vi "Display FI locations on tiled image.vi"(5 "[user-specified font]":T1={"Font Name:"="", "Size"=8, "Strikeout?"=FALSE, "Italic?"=FALSE, "Underline?"=FALSE, "Outline?"=FALSE, "Shadow?"=FALSE, "Bold?"=FALSE}, 6 "Symbol":string="+", 7 "Primary grid @ green":bool=TRUE, 8 "Tiled Image fit to":u8(ring) items=["Width", "Height"], 9 "Focus Index Options":T2={"Keep aspect ratio"=FALSE, "Show Focus Index"=TRUE, "Focus Index primary grid center"=TRUE, "X Grids"=[[1]], "Y Grids"=[[1]], "Primary X index"=[[1]], "Primary Y index"=[[1]]} {"Y Grids" step=2; "X Grids" step=2}, 10 "SEM Scan Parameters":T3={"X size (um)"=80.0, "Y size (um)"=80.0, "X center (um)"=0.0, "Y center (um)"=0.0, "X size (V)"=3.7333333333333334, "X size auto"=TRUE, "X stig"=[[0.0]], "Y stig"=[[0.0]], "X aln"=[[0.0]], "Y aln"=[[0.0]], "Scan rate (Hz)"=10000000, "Oversampling"=5, "Oversampling auto"=TRUE, "Frame line rampdown ratio"=0.1, "Pixel size (nm)"=8.0, "WD (mm)"=[[3.0]], "X tiles"=1, "Y tiles"=1, "Overlap (um)"=2.0, "Interlaced"=TRUE, "dX (um)"=[0.0], "dY (um)"=[0.0], "Frames"=1} {"dY (um)" format="%.1f"; "dX (um)" format="%.1f"; "Frames" min=1 step=1; "WD (mm)" step=0.001 format="%.4f"; "Y aln" format="%.1f"; "X aln" format="%.1f"; "Y stig" format="%.1f"; "X stig" format="%.1f"; "Overlap (um)" min=0; "Y tiles" min=1; "X tiles" min=1; "X size (um)" format="%.2f"; "Y size (um)" format="%.2f"; "Frame line rampdown ratio" min=0 max=1 step=0.05 format="%.2g"; "X center (um)" step=1 format="%.3f"; "Y center (um)" step=1 format="%.3f"; "X size (V)" format="%_4g"; "Scan rate (Hz)" max=4000000 step=100000 format="%.2e"}, 11 "Image reference":refnum<vi>) -> ()   [LabVIEW 2018]
panel:
  # "Grids"
  # "Primary"
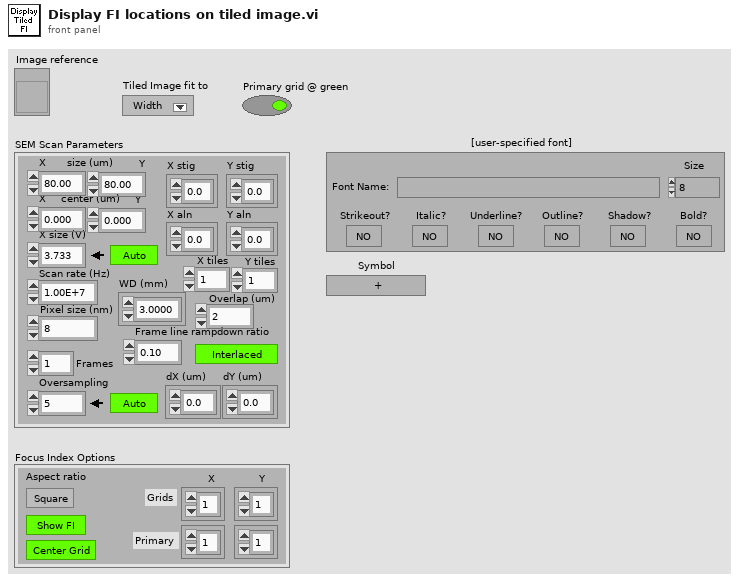
[diagram p1: front panel]
types:
  T1 = cluster{"Font Name:":string, "Size":i16, "Strikeout?":bool, "Italic?":bool, "Underline?":bool, "Outline?":bool, "Shadow?":bool, "Bold?":bool}
  T2 = cluster{"Keep aspect ratio":bool, "Show Focus Index":bool, "Focus Index primary grid center":bool, "X Grids":u8[][], "Y Grids":u8[][], "Primary X index":u8[][], "Primary Y index":u8[][]}
  T3 = cluster{"X size (um)":sgl, "Y size (um)":sgl, "X center (um)":sgl, "Y center (um)":sgl, "X size (V)":dbl, "X size auto":bool, "X stig":sgl[][], "Y stig":sgl[][], "X aln":sgl[][], "Y aln":sgl[][], "Scan rate (Hz)":u32, "Oversampling":u32, "Oversampling auto":bool, "Frame line rampdown ratio":sgl, "Pixel size (nm)":sgl, "WD (mm)":sgl[][], "X tiles":u8, "Y tiles":u8, "Overlap (um)":sgl, "Interlaced":bool, "dX (um)":sgl[], "dY (um)":sgl[], "Frames":u8}
  T4 = cluster{"horizontal":enum16{"left", "center", "right"}, "vertical":enum16{"top", "center", "bottom"}}
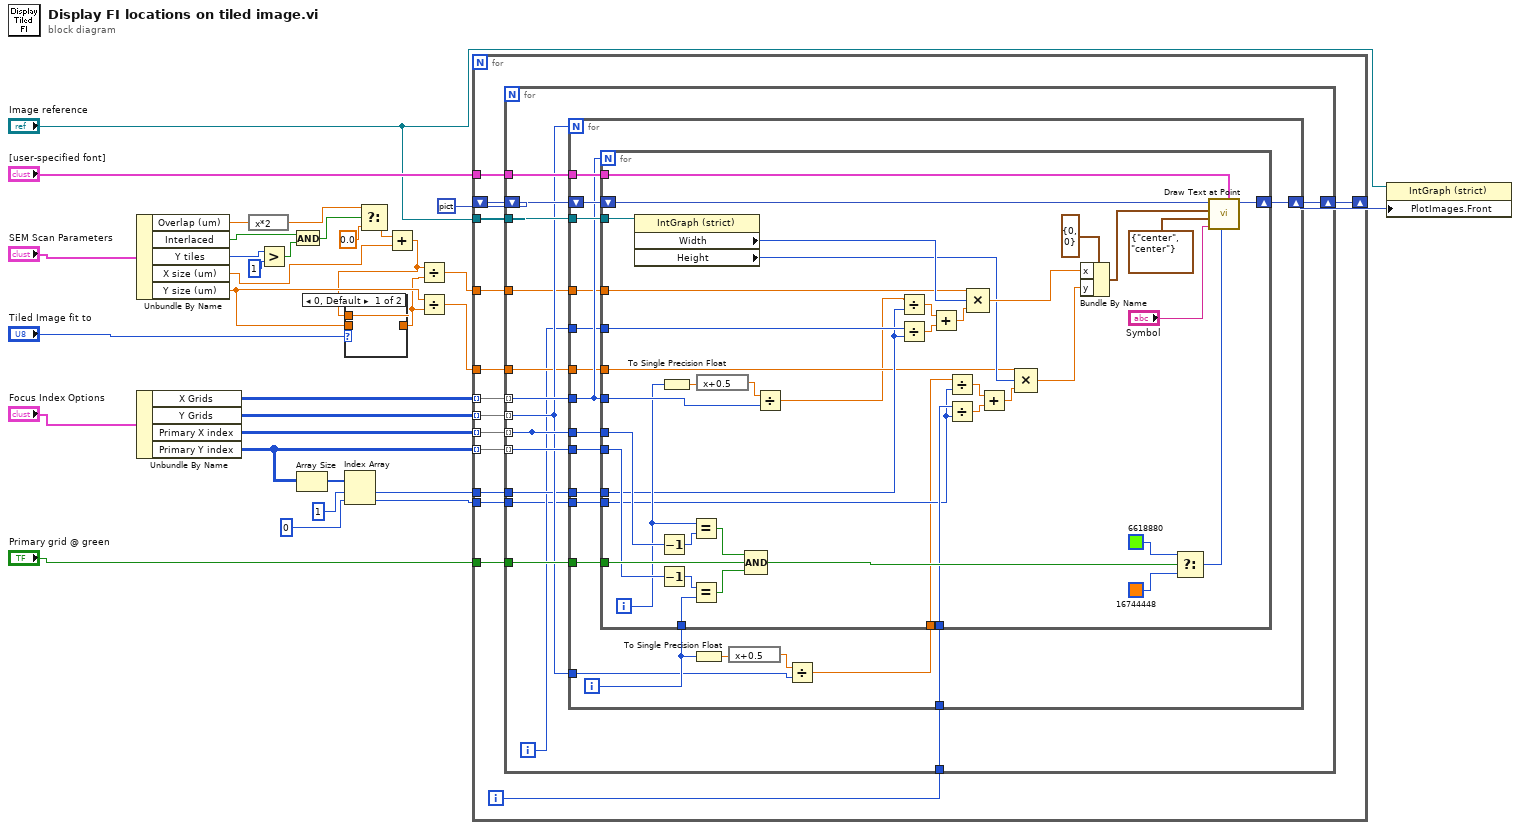
[diagram p0: block diagram]
diagram:
  n1 = Unbundle By Name("SEM Scan Parameters") -> ("Overlap (um)"=w7:sgl, "Interlaced"=w2:bool, "Y tiles"=w5:u8, "X size (um)"=w11:sgl, "Y size (um)"=w23:sgl)
  n2 = Unbundle By Name("Focus Index Options") -> ("X Grids"=w30:u8[][], "Y Grids"=w29:u8[][], "Primary X index"=w27:u8[][], "Primary Y index"=w16:u8[][])
  n3 = expression code="x*2"(w7) -> (w8:sgl)
  n4 = Greater?(x=w5, y=u8 1) -> (0:w3:bool)
  n5 = And(x=w2, y=w3) -> (x .and. y?=w1:bool)
  n6 = Array Size(array=w16) -> (size(s)=w17:i32[])
  n7 = Index Array(array=w17, index #1=1 ("index"), index #2=0 ("index")) -> (element #1=w15:i32, element #2=w14:i32)
  n8 = Select(t=w8, s=w1, f=0.0) -> (s? t:f=w10:dbl)
  n9 = Add(x=w10, y=w11) -> (x+y=w6:dbl)
  n10 = case shown="0, Default" "Tiled Image fit to" {
    tunnel: w6 -> [w33 _]
    tunnel: w23 -> [_ w34]
    tunnel: [w33 w34] -> w22
    frame 0, Default {
    }
    frame 1 {
    }
  }
  n11 = Divide(x=w6, y=w22) -> (x/y=w21:dbl)
  n12 = Divide(x=w23, y=w22) -> (x/y=w20:dbl)
  n13 = for {
    tunnel: w30 -> [w48] mode=indexing
    tunnel: w29 -> [w47] mode=indexing
    tunnel: "Image reference" -> [w46]
    shift-right: [w45] -> w13
    shift-left: picture data[5B] ("picture") -> [w44]
    tunnel: w27 -> [w43] mode=indexing
    tunnel: w16 -> [w42] mode=indexing
    tunnel: "[user-specified font]" -> [w41]
    tunnel: "Primary grid @ green" -> [w40]
    tunnel: w21 -> [w39]
    tunnel: w20 -> [w38]
    tunnel: w15 -> [w37]
    tunnel: w14 -> [w36]
    i -> [w35]
    n14 = for {
      tunnel: w48 -> [w63] mode=indexing
      tunnel: w47 -> [w55] mode=indexing
      tunnel: w46 -> [w62]
      shift-right: [w61] -> w45
      shift-left: w44 -> [w60]
      tunnel: [w57] -> _ mode=indexing
      tunnel: w43 -> [w57] mode=indexing
      tunnel: w42 -> [w56] mode=indexing
      tunnel: w41 -> [w59]
      tunnel: w40 -> [w58]
      tunnel: w39 -> [w54]
      tunnel: w38 -> [w53]
      tunnel: w37 -> [w52]
      tunnel: w36 -> [w50]
      tunnel: w35 -> [w49]
      i -> [w51]
      n15 = for {
        N: w55 -> [_]
        tunnel: w63 -> [w71]
        tunnel: w62 -> [w82]
        shift-right: [w81] -> w61
        shift-left: w60 -> [w80]
        tunnel: w59 -> [w79]
        tunnel: w58 -> [w78]
        tunnel: w57 -> [w77]
        tunnel: w56 -> [w76]
        tunnel: w55 -> [w72]
        tunnel: w54 -> [w70]
        tunnel: w53 -> [w68]
        tunnel: w52 -> [w67]
        tunnel: w51 -> [w66]
        tunnel: w50 -> [w65]
        tunnel: w49 -> [w64]
        i -> [w73]
        n16 = To Single Precision Float(number=w73) -> (single precision float=w74:sgl)
        n17 = expression code="x+0.5"(w74) -> (w75:sgl)
        n18 = Divide(x=w75, y=w72) -> (x/y=w69:sgl)
        n19 = for {
          N: w71 -> [_]
          tunnel: w82 -> [w121]
          shift-right: [w120] -> w81
          shift-left: w80 -> [w119]
          tunnel: w79 -> [w118]
          tunnel: w73 -> [w108]
          tunnel: w78 -> [w107]
          tunnel: w77 -> [w106]
          tunnel: w76 -> [w105]
          tunnel: w71 -> [w102]
          tunnel: w70 -> [w83]
          tunnel: w69 -> [w86]
          tunnel: w68 -> [w85]
          tunnel: w67 -> [w98]
          tunnel: w66 -> [w99]
          tunnel: w65 -> [w88]
          tunnel: w64 -> [w89]
          i -> [w101]
          n20 = property on="Property Node" class="IntGraph (strict)"(reference=w121) -> ("Width"=w95:u32, "Height"=w90:u32)  [unwired: 1 in, 2 out]
          n21 = Decrement(x=w106) -> (x-1=w112:u8)
          n22 = Decrement(x=w105) -> (x-1=w113:u8)
          n23 = To Single Precision Float(number=w101) -> (single precision float=w104:sgl)
          n24 = Equal?(x=w101, y=w112) -> (x = y?=w111:bool)
          n25 = Equal?(x=w113, y=w108) -> (x = y?=w110:bool)
          n26 = expression code="x+0.5"(w104) -> (w103:sgl)
          n27 = Compound Arithmetic op=AND(w111, w107, w110) -> (w109:bool)
          n28 = Divide(x=w103, y=w102) -> (x/y=w84:sgl)
          n29 = Divide(x=w84, y=w98) -> (x/y=w100:sgl)
          n30 = Divide(x=w99, y=w98) -> (x/y=w97:dbl)
          n31 = Add(x=w100, y=w97) -> (x+y=w96:dbl)
          n32 = Divide(x=w86, y=w88) -> (x/y=w91:sgl)
          n33 = Divide(x=w89, y=w88) -> (x/y=w92:dbl)
          n34 = Compound Arithmetic op=MULTIPLY(w83, w95, w96) -> (w94:dbl)
          n35 = Add(x=w91, y=w92) -> (x+y=w93:dbl)
          n36 = Compound Arithmetic op=MULTIPLY(w85, w90, w93) -> (w87:dbl)
          n37 = Bundle By Name(cluster=cluster{"x":i16, "y":i16} {"x"=0, "y"=0} ("origin"), "x"=w94, "y"=w87) -> (w122:cluster{"x":i16, "y":i16})
          n38 = Select(t=u32 6618880 ("text color(black)"), s=w109, f=u32 16744448 ("text color(black)")) -> (s? t:f=w114:u32)
          n39 = call <vilib>:"Draw Text at Point.vi"("[user-specified font]"=w118, "text color(black)"=w114, "text"="Symbol", "alignment(left, top)"=T4 {"horizontal"=enum."center", "vertical"=enum."center"}, "origin"=w122, "picture"=w119) -> ("new picture"=w120:picture)  [unwired: 4 in, 1 out]
        }
      }
    }
  }
  n40 = property on="Property Node" class="IntGraph (strict)"(reference="Image reference", "PlotImages.Front"=w13) -> ()  [unwired: 1 in, 2 out]
